vi "getSunplusSocketVendor.vi"(10 "Device":string="QDY494") -> (2 "Vendor":string)   [LabVIEW 2012]
uses:
  <vilib>/addons/database/Connection.llb/DB Tools Open Connec (Path).vi
  <vilib>/addons/database/Connection.llb/Conn Execute.vi
  <vilib>/addons/database/Recordset.llb/Rec Fetch String Data (R).vi
  <vilib>/addons/database/Recordset.llb/Rec Destroy - Connection.vi
  <vilib>/addons/database/NI_Database_API.lvlib
panel:
  out "concatenated string":string
  out "error out":errorcluster
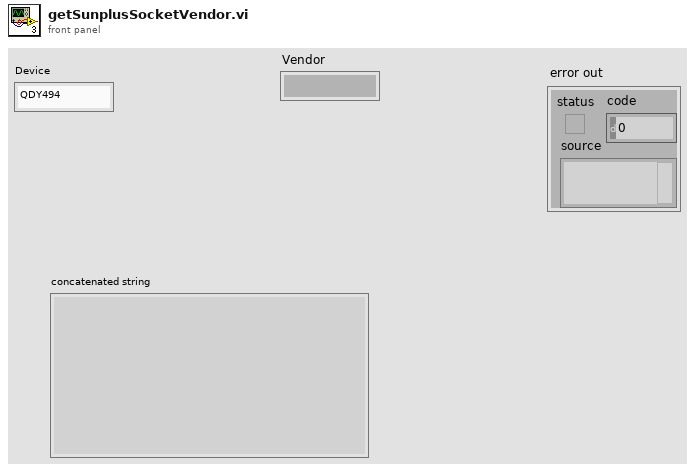
[diagram p1: front panel]
types:
  T1 = typedef "NI_Database_API.lvlib/Conn ObjectReference.ctl" = refnum<k1>
  T2 = typedef "NI_Database_API.lvlib/Rec ObjectReference.ctl" = refnum<k1>
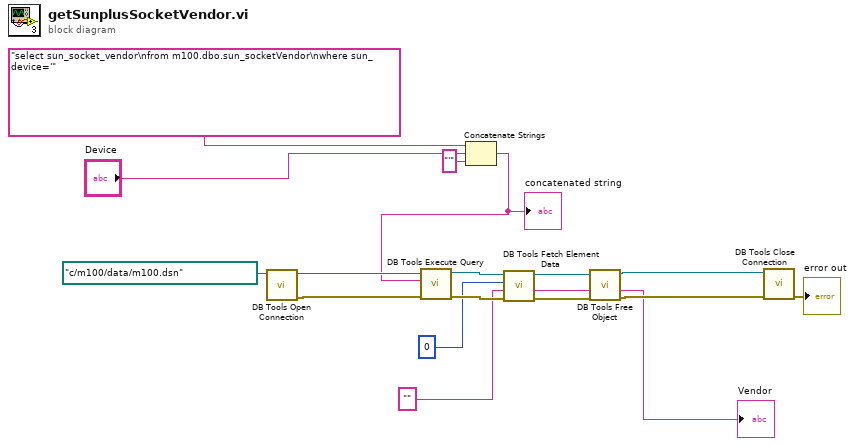
[diagram p0: block diagram]
diagram:
  n1 = call-poly <vilib>:"DB Tools Open Connection.vi"("connection information"=path "c:/m100/data/m100.dsn") -> ("error out"=w11:errorcluster, "connection reference"=w12:T1)  [unwired: 7 in]
  n2 = Concatenate Strings("select sun_socket_vendor\nfrom m100.dbo.sun_socketVendor\nwhere sun_device='" ("SQL query"), "Device", "'" ("string")) -> (w4:string)
  "concatenated string" <- w4
  n3 = call-poly <vilib>:"DB Tools Execute Query.vi"("error in (no error)"=w11, "SQL query"=w4, "connection reference"=w12) -> ("error out"=w17:errorcluster, "recordset reference"=w16:T2)  [unwired: 5 in]
  n4 = call-poly <vilib>:"DB Tools Fetch Element Data.vi"("error in (no error)"=w17, "type"="", "column index"=0, "recordset reference"=w16) -> ("error out"=w14:errorcluster, "data"=→"Vendor":string, "recordset reference out"=w15:T2)  [unwired: 3 in]
  n5 = call-poly <vilib>:"DB Tools Free Object.vi"("error in (no error)"=w14, "recordset reference"=w15) -> ("error out"=w9:errorcluster, "connection reference"=w10:T1)  [unwired: 8 in]
  n6 = call <vilib>:"DB Tools Close Connection.vi"("error in (no error)"=w9, "connection reference"=w10) -> ("error out"=→"error out":errorcluster)  [unwired: 5 in]
